vi "Log Event.vi"(8 "error in":errorcluster, 10 "event":string, 11 "module reference in":T1) -> (0 "error out":errorcluster, 3 "module reference out":T1)   [LabVIEW 2017, in "Logger.lvlib"]
uses:
  Logger.lvlib
  Private TypeDefs/Module Reference.ctl
  Global TypeDefs/Registered Modules.ctl
  Private TypeDefs/Module Queues.ctl
  Private TypeDefs/Message Queue Element.ctl
  Private TypeDefs/Messages.ctl
  Private TypeDefs/Module Notifiers.ctl
  Private TypeDefs/Dummy Notifier.ctl
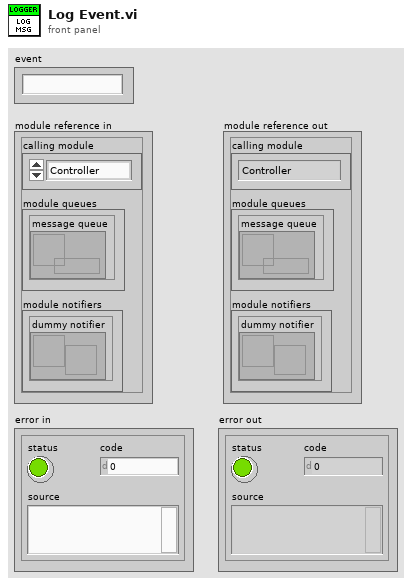
[diagram p1: front panel]
types:
  T1 = typedef "Logger.lvlib/Module Reference.ctl" = cluster{"calling module":T2, "module queues":T3, "module notifiers":T4}
  T2 = typedef "Registered Modules.ctl" = enum16{"Controller", "DAQ", "Error Handler", "Game", "myPAM", "WinHost", "Logger"}
  T3 = typedef "Logger.lvlib/Module Queues.ctl" = cluster{"message queue":refnum<queue>}
  T4 = typedef "Logger.lvlib/Module Notifiers.ctl" = cluster{"dummy notifier":refnum<notifier>}
  T5 = typedef "Logger.lvlib/Message Queue Element.ctl" = cluster{"source":T2, "message":T6, "data":variant}
  T6 = typedef "Logger.lvlib/Messages.ctl" = enum16{"log event", "shutdown"}
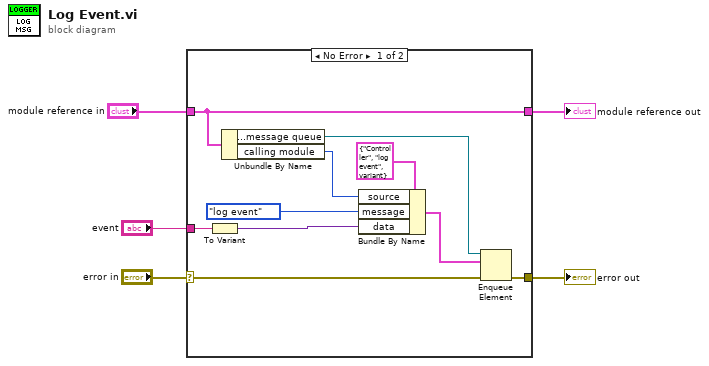
[diagram p0: block diagram]
diagram:
  n1 = case shown="No Error" "error in" {
    selector: "error in" -> [w14 w17]
    tunnel: [w13 w17] -> w4
    tunnel: "event" -> [w11 _]
    tunnel: "module reference in" -> [w7 w16]
    tunnel: [w7 w16] -> w1
    frame No Error {
      n2 = To Variant(anything=w11) -> (Variant=w12:variant)
      n3 = Unbundle By Name(w7) -> ("module queues.message queue"=w8:refnum<queue>, "calling module"=w6:T2)
      n4 = Bundle By Name(cluster=T5 {"source"=enum."Controller", "message"=enum."log event", "data"=variant} ("message queue element"), "source"=w6, "message"=Messages."log event" ("messages"), "data"=w12) -> (w15:T5)
      n5 = Enqueue Element(queue=w8, element=w15, error in (no error)=w14) -> (error out=w13:errorcluster)  [unwired: 1 in, 2 out]
    }
    frame Error {
    }
  }
  "error out" <- w4
  "module reference out" <- w1
